vi "read_burstData.vi"(8 "error in":errorcluster, 11 "DirPath":path) -> (0 "error out":errorcluster, 2 "Specs_time":cluster{"Waveform":waveform(dbl), timestamp}[](array[cluster]), 3 "Specs":dbl[][](graph))   [LabVIEW 2016]
uses:
  Tools/Intensity_rainbow_pattern.ctl
  <vilib>/Analysis/baseanly.llb/Mean (DBL).vi
  <vilib>/addons/Digital Filter Design/Design.llb/DFD IIR Notch Peak Design by BW.vi
  <vilib>/addons/Digital Filter Design/Process.llb/DFD Filtering (Array NChan).vi
  <vilib>/Analysis/NI_AALPro.lvlib
  <vilib>/addons/Digital Filter Design/NI_DigFilterLicensed.lvlib
  <vilib>/Analysis/NI_AALBase.lvlib
panel:
  out "Comp":waveform(dbl)[](graph)
  out "Filter":waveform(dbl)[](graph)
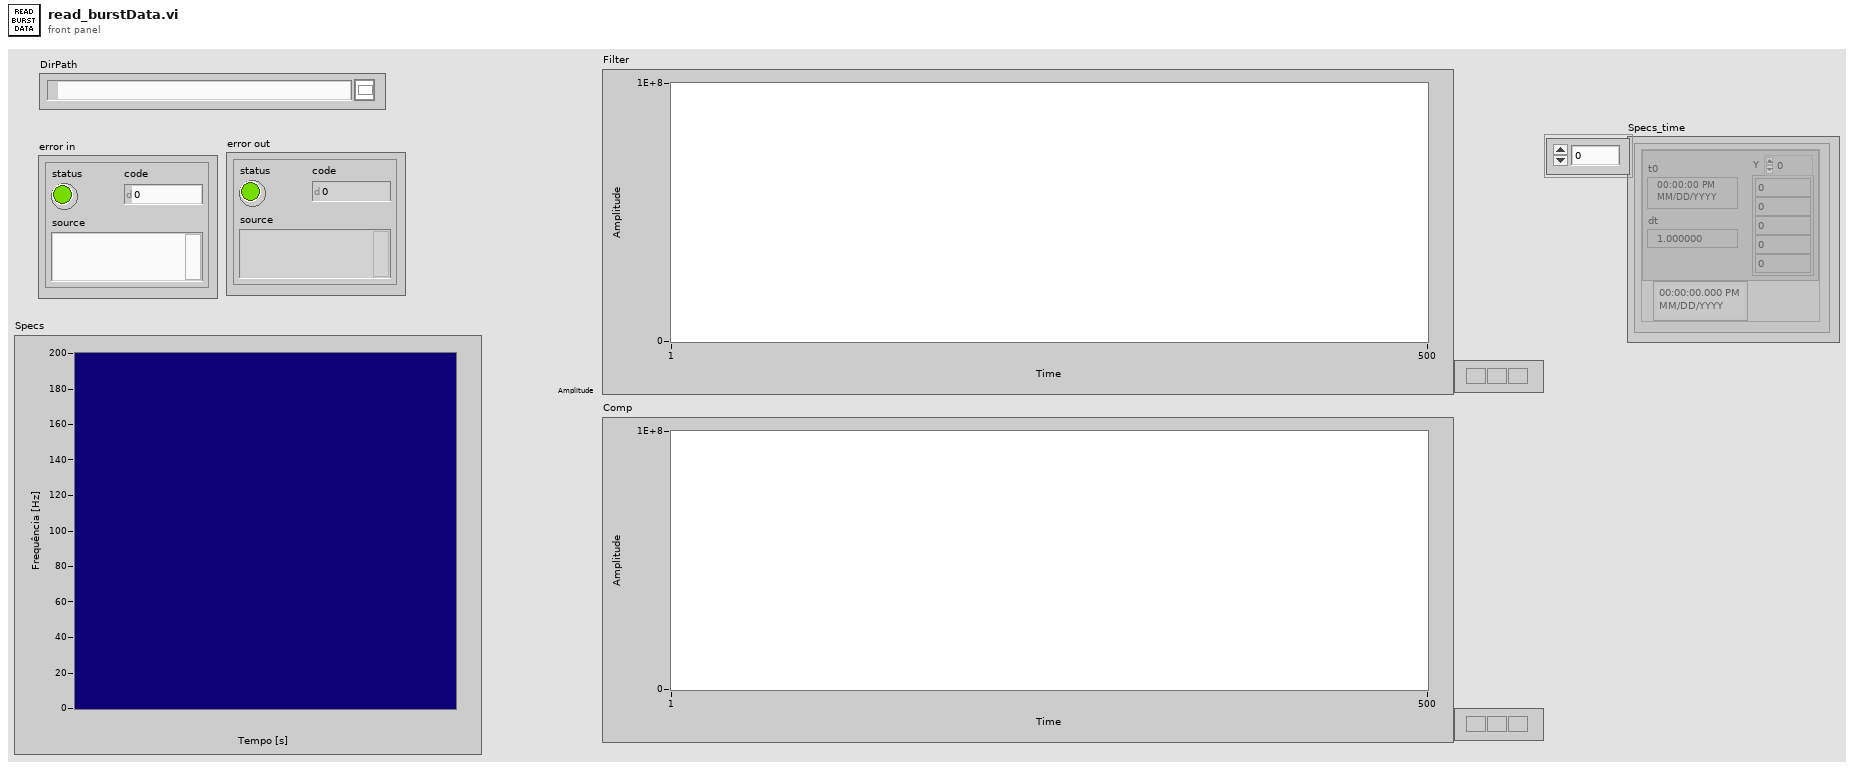
[diagram p1: front panel]
types:
  T1 = typedef "Intensity_rainbow_pattern.ctl" = u32[]
  T2 = typedef "NI_DigFilterLicensed.lvlib/DFD Filter Obj.ctl" = cluster{"mSRate_Fs":dbl, "mSRate_Version":string, "mSRate_Comments":string, "mSRate_OrgCoef":T3, "mSRate_CurCoef":T3, "mSRate_Quantized?":bool, "mSRate_QCoef":T3, "mSRate_QSettings":T5[], "mSRate_Order":i32, "mSRate_Scaling":cluster{"mSRate_ScaleByPowerOf2?":bool, "mSRate_ScaleType":T7}}
  T3 = typedef "NI_DigFilterLicensed.lvlib/DFD Filter Coef.ctl" = cluster{"type":T4, "gain":dbl, "coef a (k)":dbl[], "coef b (v)":dbl[]}
  T4 = typedef "NI_DigFilterLicensed.lvlib/DFD Filter Structure Type Selector.ctl" = enum16{"Undefined", "FIR Direct Form", "FIR Direct Form Transposed", "FIR Symmetric", "FIR Antisymmetric", "IIR Direct Form I", "IIR Direct Form I Transposed", "IIR Direct Form II", "IIR Direct Form II Transposed", "IIR Cascaded Second Order Sections Form I", "IIR Cascaded Second Order Sections Form I Transposed", "IIR Cascaded Second Order Sections Form II", "IIR Cascaded Second Order Sections Form II Transposed", "Lattice Allpass (basic sections)", "Lattice Allpass (one multiplier sections)", "Lattice Allpass (normalized sections)", "Lattice AR (basic sections)", "Lattice AR (one multiplier sections)", "Lattice AR (normalized sections)", "Lattice MA (minimum phase)", "Lattice MA (maximum phase)", "Lattice ARMA (basic sections)", "Lattice ARMA (one multiplier sections)", "Lattice ARMA (normalized sections)"}
  T5 = typedef "NI_DigFilterLicensed.lvlib/dfd_Internal Quantization Settings.ctl" = cluster{"source":T6, "wl":i16, "iwl":i16, "overflow mode":enum16{"Saturation", "Wrap"}, "rounding mode":enum16{"Nearest", "Truncation"}, "signed?":bool}
  T6 = typedef "NI_DigFilterLicensed.lvlib/dfd_Internal Quantization Srcs.ctl" = u16
  T7 = typedef "NI_DigFilterLicensed.lvlib/DFD Coef Norm Type.ctl" = enum16{"No Norm", "Time Domain 1-Norm", "Time Domain 2-Norm", "Time Domain Inf-Norm"}
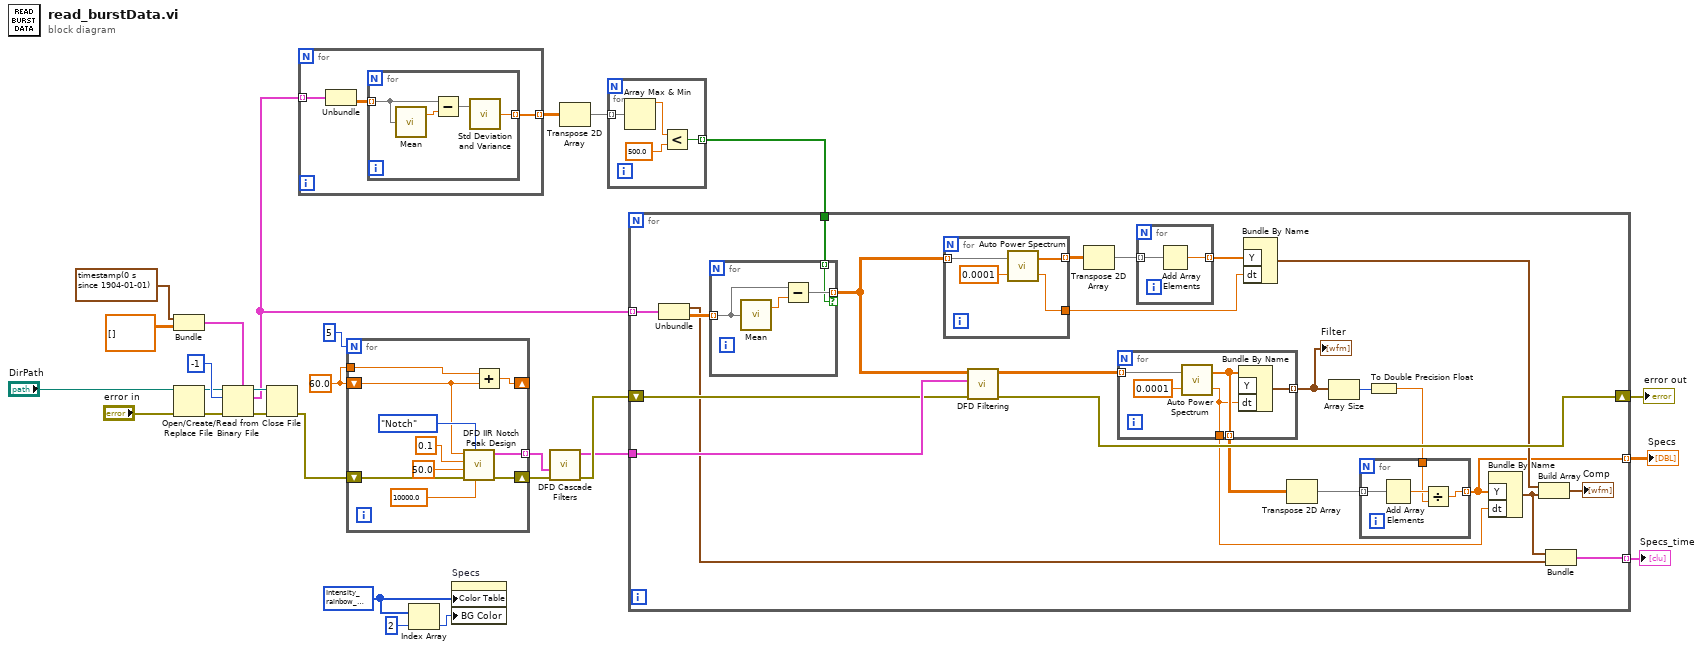
[diagram p0: block diagram]
diagram:
  w6 = T1 [786534, 852078, 917622, 983166, 1048710, 1114254, 1179798, 1245342, 1310886, 1376430, 1376439, 1441983, 1507527, 1573071, 1638615, 1704159, 1769703, 1835247, 1900791, 1966335, 1966335, 1835263, 1638655, 1507583, 1310975, 1179903, 983295, 852223, 655615, 524543, 327935, 196863, 511, 1791, 3071, 4351, 5631, 6911, 8191, 9471, 10751, 12031, 13311, 14591, 15871, 17151, 18431, 19711, 20991, 22271, 23551, 24831, 26111, 27391, 28671, 29951, 31231, 32511, 33791, 35071, 36351, 37631, 38911, 40191, 41471, 42751, 44031, 45311, 46591, 47871, 49151, 50431, 51711, 52991, 54271, 55551, 56831, 58111, 59391, 60671, 61951, 63231, 64511, 65532, 65527, 65522, 65517, 65512, 65507, 65502, 65497, 65492, 65487, 65482, 65477, 65472, 65467, 65462, 65457, 65452, 65447, 65442, 65437, 65432, 65427, 65422, 65417, 65412, 65407, 65402, 65397, 65392, 65387, 65382, 65377, 65372, 65367, 65362, 65357, 65352, 65347, 65342, 65337, 65332, 65327, 65322, 65317, 65312, 65307, 65302, 65297, 65292, 65287, 65282, 261888, 589568, 917248, 1244928, 1572608, 1900288, 2227968, 2555648, 2883328, 3211008, 3538688, 3866368, 4194048, 4521728, 4849408, 5177088, 5504768, 5832448, 6160128, 6487808, 6815488, 7143168, 7470848, 7798528, 8126208, 8453888, 8781568, 9109248, 9436928, 9764608, 10092288, 10419968, 10747648, 11075328, 11403008, 11730688, 12058368, 12386048, 12713728, 13041408, 13369088, 13696768, 14024448, 14352128, 14679808, 15007488, 15335168, 15662848, 15990528, 16318208, 16645888, 16775936, 16774656, 16773376, 16772096, 16770816, 16769536, 16768256, 16766976, 16765696, 16764416, 16763136, 16761856, 16760576, 16759296, 16758016, 16756736, 16755456, 16754176, 16752896, 16751616, 16750336, 16749056, 16747776, 16746496, 16745216, 16743936, 16742656, 16741376, 16740096, 16738816, 16737536, 16736256, 16734976, 16733696, 16732416, 16731136, 16729856, 16728576, 16727296, 16726016, 16724736, 16723456, 16722176, 16720896, 16719616, 16718336, 16717056, 16715776, 16714496, 16713216, 16711680, 16711680, 16449536, 16187392, 15925248, 15663104, 15400960, 15138816, 14876672, 14614528, 14352384, 14090240, 13828096, 13565952, 13303808, 13041664, 12779520, 12517376, 12255232, 11993088, 11665408] ("Rainbow pattern Sirino")
  w16 = 60.0 ("f0 [Hz]")
  n1 = Bundle(timestamp(0 s since 1904-01-01), dbl[][] []) -> (w27:cluster{timestamp, dbl[][]})  [unwired: 1 in]
  n2 = Open/Create/Replace File(file path (use dialog)="DirPath", error in="error in") -> (refnum out=w20:refnum<file>, error out=w21:errorcluster)  [unwired: 4 in, 1 out]
  n3 = Read from Binary File(5:w27, 8:w21, 10:-1 ("count (1)"), 11:w20) -> (0:w24:errorcluster, 2:w5:cluster{timestamp, dbl[][]}[], 3:w23:refnum<file>)  [unwired: 2 in, 1 out]
  n4 = Close File(refnum=w23, error in=w24) -> (error out=w15:errorcluster)  [unwired: 1 out]
  n5 = for {
    tunnel: w5 -> [w29] mode=indexing
    tunnel: [w28] -> w4 mode=indexing
    n6 = Unbundle(w29) -> (w30:dbl[][])  [unwired: 1 out]
    n7 = for {
      tunnel: w30 -> [w32] mode=indexing
      tunnel: [w34] -> w28 mode=indexing
      n8 = call-poly <vilib>:"Mean.vi"("X"=w32) -> ("mean"=w33:dbl)  [unwired: 1 out]
      n9 = Subtract(x=w32, y=w33) -> (x-y=w31:dbl[])
      n10 = call <vilib>:"Std Deviation and Variance.vi"("X"=w31) -> ("standard deviation"=w34:dbl)  [unwired: 1 in, 2 out]
    }
  }
  n11 = for {
    N: 5 -> [_]
    tunnel: [w41] -> w14 mode=indexing
    shift-right: [w38] -> _
    shift-left: w16 -> [w37]
    tunnel: w16 -> [w39]
    shift-right: [w35] -> w13
    shift-left: w15 -> [w36]
    n12 = call-poly <vilib>:"DFD IIR Notch Peak Design.vi"("fs [Hz]"=10000.0, "filter type"=enum16{"Notch", "Peak"}."Notch", "error in (no error)"=w36, "Ab [dB]"=50.0, "Df [Hz]"=0.1, "f0 [Hz]"=w37) -> ("error out"=w35:errorcluster, "filter out"=w41:T2)  [unwired: 4 in]
    n13 = Add(x=w39, y=w37) -> (x+y=w38:dbl)
  }
  n14 = Index Array(array=w6, index=2) -> (element=w8:u32)
  n15 = property on="Specs" class="IntGraph (strict)"("Color Table"=w6, "BG Color"=w8) -> ()  [unwired: 2 in, 2 out]
  n16 = call <vilib>:"DFD Cascade Filters.vi"("error in (no error)"=w13, "filters in"=w14) -> ("error out"=w12:errorcluster, "filter out"=w11:T2)  [unwired: 8 in]
  n17 = Transpose 2D Array(2D array=w4) -> (transposed array=w3:dbl[][])
  n18 = for {
    tunnel: w3 -> [w46] mode=indexing
    tunnel: [w47] -> w2 mode=indexing
    n19 = Array Max & Min(array=w46) -> (max value=w45:dbl)  [unwired: 3 out]
    n20 = Less?(x=w45, y=500.0) -> (x < y?=w47:bool)
  }
  n21 = for {
    tunnel: w5 -> [w72] mode=indexing
    tunnel: w11 -> [w71]
    shift-right: [w69] -> w10
    shift-left: w12 -> [w70]
    tunnel: [w56] -> w9 mode=indexing
    tunnel: w2 -> [w55]
    tunnel: [w52] -> w1 mode=indexing
    n22 = Unbundle(w72) -> (w53:timestamp, w67:dbl[][])
    n23 = for {
      tunnel: w67 -> [w75] mode=indexing
      tunnel: [w74] -> w66 mode=indexing if=w73
      tunnel: w55 -> [w73] mode=indexing
      n24 = call-poly <vilib>:"Mean.vi"("X"=w75) -> ("mean"=w76:dbl)  [unwired: 1 out]
      n25 = Subtract(x=w75, y=w76) -> (x-y=w74:dbl[])
    }
    n26 = for {
      tunnel: w66 -> [w86] mode=indexing
      tunnel: [w84] -> w65 mode=indexing
      tunnel: [w83] -> w62
      n27 = call <vilib>:"Auto Power Spectrum.vi"("dt"=0.0001, "Signal (V)"=w86) -> ("df"=w83:dbl, "Power Spectrum (V^2 rms)"=w84:dbl[])
    }
    n28 = call-poly <vilib>:"DFD Filtering.vi"("error in (no error)"=w70, "filter"=w71, "signal in"=w66) -> ("error out"=w69:errorcluster, "signal out"=w68:dbl[][])  [unwired: 7 in]
    n29 = Transpose 2D Array(2D array=w65) -> (transposed array=w64:dbl[][])
    n30 = for {
      tunnel: w68 -> [w91] mode=indexing
      tunnel: [w89] -> w51 mode=indexing
      tunnel: [w88] -> w60 mode=indexing
      tunnel: [w87] -> w59
      n31 = call <vilib>:"Auto Power Spectrum.vi"("dt"=0.0001, "Signal (V)"=w91) -> ("df"=w87:dbl, "Power Spectrum (V^2 rms)"=w88:dbl[])
      n32 = Bundle By Name("Y"=w88, "dt"=w87) -> (w89:waveform(dbl))  [unwired: 1 in]
    }
    "Filter" <- w51
    n33 = for {
      tunnel: w64 -> [w82] mode=indexing
      tunnel: [w81] -> w63 mode=indexing
      n34 = Add Array Elements(numeric array=w82) -> (sum=w81:dbl)
    }
    n35 = Bundle By Name("Y"=w63, "dt"=w62) -> (w58:waveform(dbl))  [unwired: 1 in]
    n36 = Transpose 2D Array(2D array=w60) -> (transposed array=w61:dbl[][])
    n37 = Array Size(array=w51) -> (size(s)=w50:i32)
    n38 = To Double Precision Float(number=w50) -> (double precision float=w49:dbl)
    n39 = for {
      tunnel: w61 -> [w80] mode=indexing
      tunnel: [w78] -> w56 mode=indexing
      tunnel: w49 -> [w77]
      n40 = Add Array Elements(numeric array=w80) -> (sum=w79:dbl)
      n41 = Divide(x=w79, y=w77) -> (x/y=w78:dbl)
    }
    n42 = Bundle By Name("Y"=w56, "dt"=w59) -> (w54:waveform(dbl))  [unwired: 1 in]
    n43 = Build Array(w58, w54) -> (→"Comp":waveform(dbl)[])
    n44 = Bundle(w54, w53) -> (w52:cluster{waveform(dbl), timestamp})  [unwired: 1 in]
  }
  "error out" <- w10
  "Specs" <- w9
  "Specs_time" <- w1
